vi "Take_Mass_Sequence-Sequence.vi"() -> ()   [LabVIEW 2013]
uses:
  libtiepie.dll
panel:
  in  "ConfiguredLaserCom":refnum<visa-resource-name>
  in  "Coil_angle step":dbl
  in  "Coil_radius step":dbl
  out "PlatformYCoil":dbl[](array[numeric])
  out "PlatformXCoil":dbl[](array[numeric])
  in  "AccumsPerCertify":u16=100
  out "PlatformY":dbl[](array[numeric])
  out "PlatformX":dbl[](array[numeric])
  in  "Stop":bool
  in  "ShotsPerEvalua":u16=100
  in  "Mass/Time":bool
  out "TenAccumulate":cluster{"MassX":dbl[], "TenScans":sgl[]}(graph)
  out "MassX":dbl[](array[numeric])
  out "TimeX":dbl[](array[numeric])
  out "PresentShot":i32
  out "Intensity_Total":sgl[](array[numeric])
  out "Intensity_SinglePoint":sgl[](array[numeric])
  out "InitializeCardErr":errorcluster
  in  "Record Length/Samples":u64=50000
  out "TpDeviceHandle_t":u32
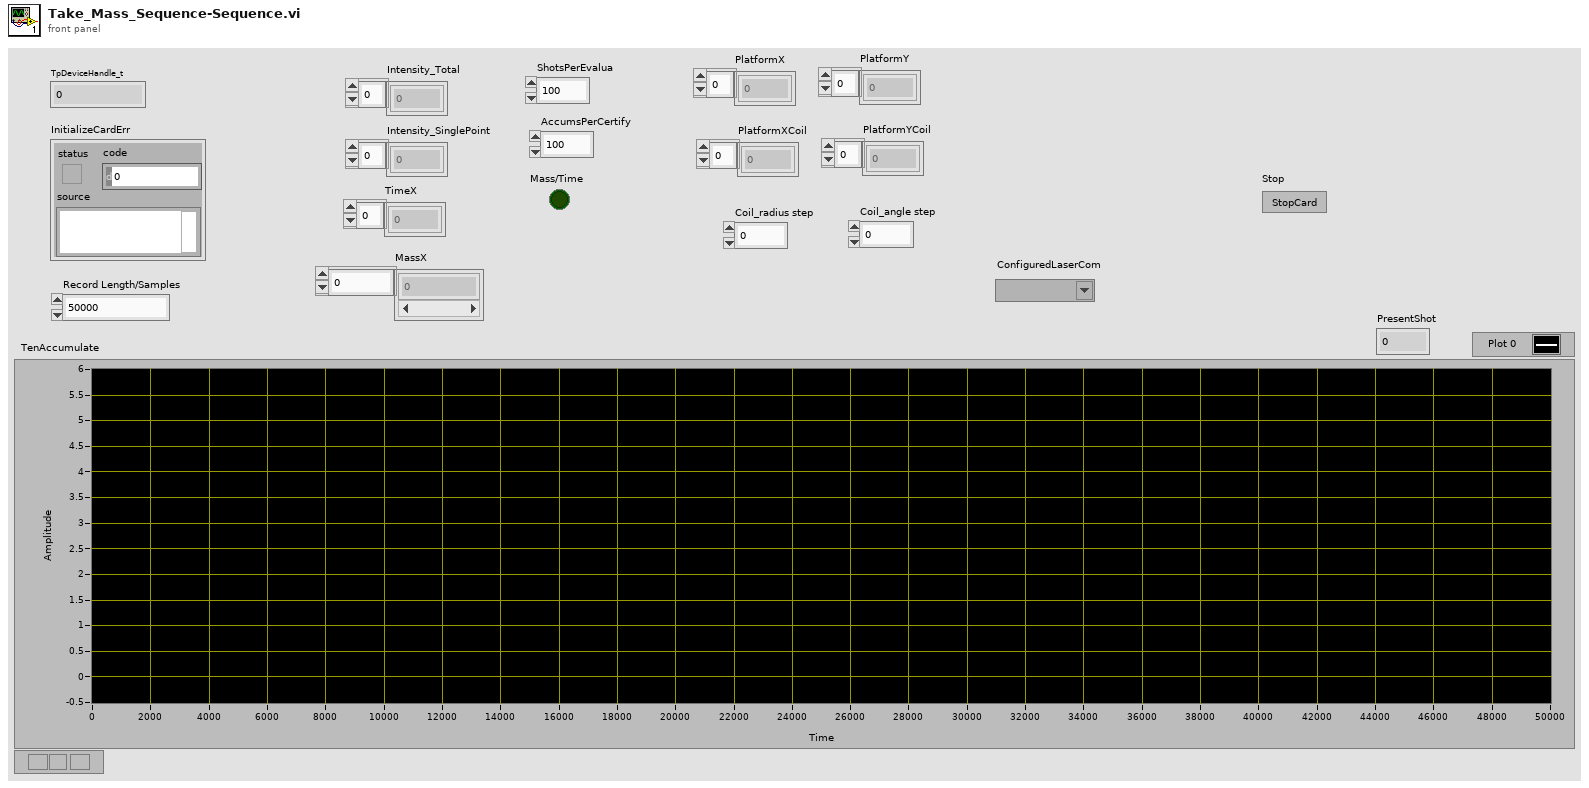
[diagram p1: front panel]
types:
  T1 = cluster{"MassX":dbl[], "Intensity_SinglePoint":sgl[]}
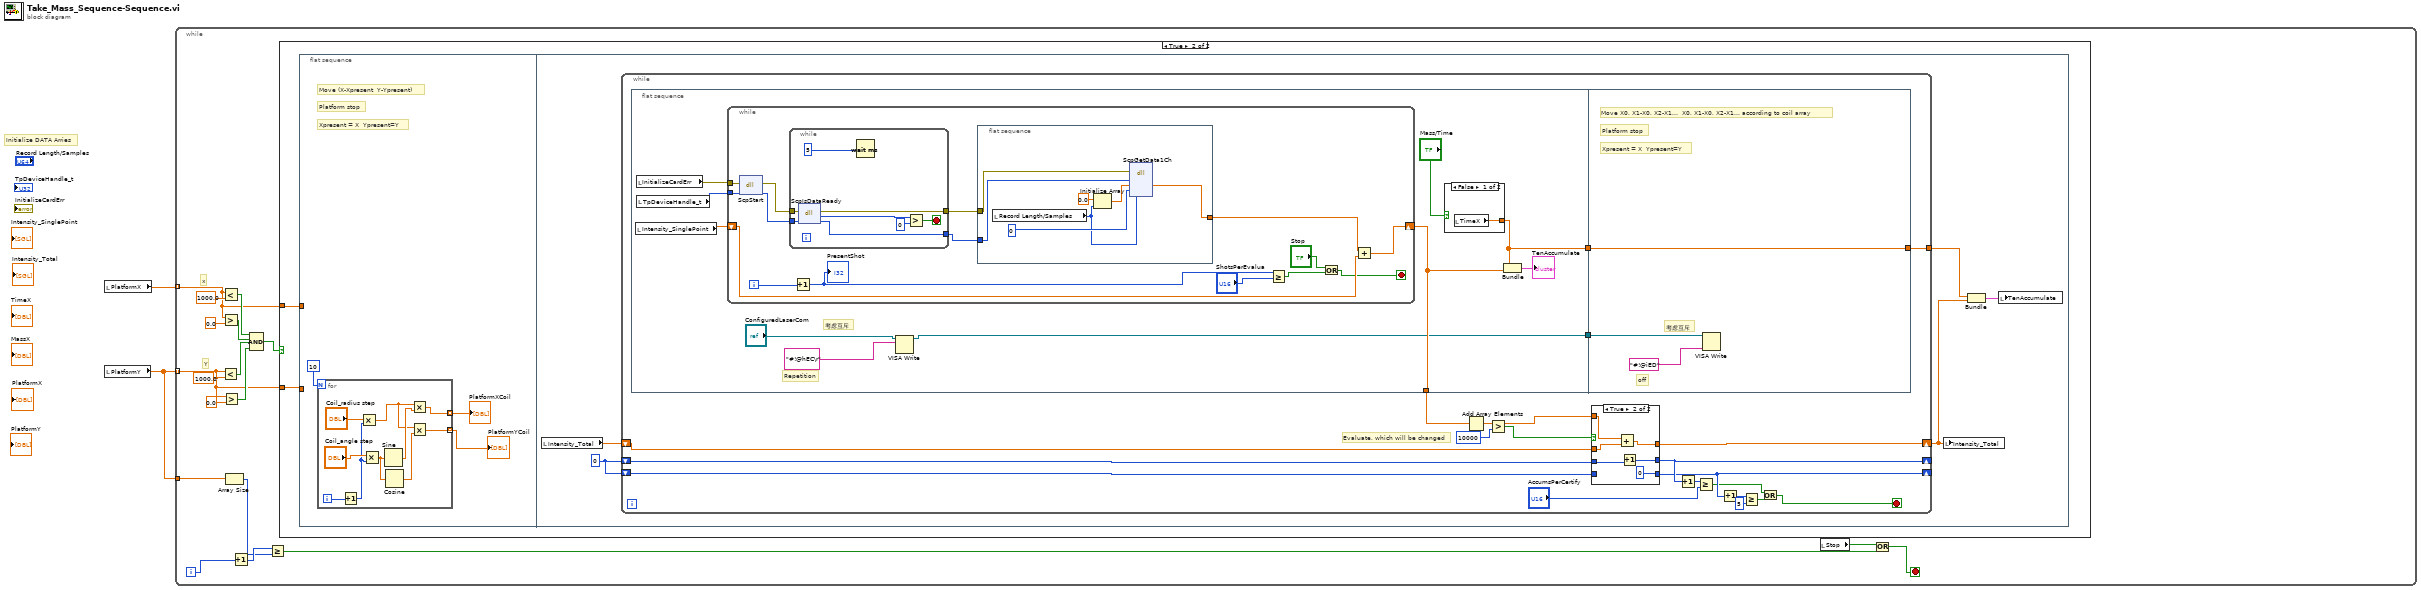
[diagram p0: block diagram]
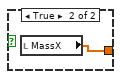
[diagram p3: hidden frame]
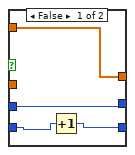
[diagram p4: hidden frame]
diagram:
  # "Initialize DATA Arries"
  n1 = local read "PlatformX"() -> (w2:dbl[])
  n2 = local read "PlatformY"() -> (w1:dbl[])
  n3 = while {
    tunnel: w2 -> [w4] mode=indexing
    tunnel: w1 -> [w3] mode=indexing
    tunnel: w1 -> [w12]
    i -> [w11]
    stop <- w6 stop-if-true
    # "Y"
    # "x"
    n4 = Less?(x=w3, y=1000.0) -> (x < y?=w14:bool)
    n5 = Less?(x=w4, y=1000.0) -> (x < y?=w16:bool)
    n6 = Greater?(x=w4, y=0.0) -> (0:w15:bool)
    n7 = Greater?(x=w3, y=0.0) -> (0:w13:bool)
    n8 = Array Size(array=w12) -> (size(s)=w9:i32)
    n9 = Increment(x=w11) -> (x+1=w10:i32)
    n10 = Compound Arithmetic op=AND(w16, w15, w14, w13) -> (w5:bool)
    n11 = Greater Or Equal?(x=w10, y=w9) -> (x >= y?=w7:bool)
    n12 = case shown="True" w5 {
      tunnel: w4 -> [_ w22]
      tunnel: w3 -> [_ w21]
      frame False {
      }
      frame True {
        n13 = flat-sequence {
          tunnel: w22 -> [_]
          tunnel: w21 -> [_]
          frame #0 {
            # "Xpresent = X  Ypresent=Y"
            # "Platform stop"
            # "Move (X-Xpresent  Y-Ypresent)"
            n14 = for {
              N: 10 -> [_]
              tunnel: [w27] -> w25 mode=indexing
              tunnel: [w26] -> w24 mode=indexing
              i -> [w35]
              n15 = Increment(x=w35) -> (x+1=w32:i32)
              n16 = Multiply(x="Coil_radius step", y=w32) -> (x*y=w28:dbl)
              n17 = Multiply(x="Coil_angle step", y=w32) -> (x*y=w31:dbl)
              n18 = Sine(x=w31) -> (sin(x)=w30:dbl)
              n19 = Cosine(x=w31) -> (cos(x)=w29:dbl)
              n20 = Multiply(x=w28, y=w30) -> (x*y=w27:dbl)
              n21 = Multiply(x=w28, y=w29) -> (x*y=w26:dbl)
            }
            "PlatformXCoil" <- w25
            "PlatformYCoil" <- w24
          }
          frame #1 {
            w39 = 0
            n22 = local read "Intensity_Total"() -> (w40:sgl[])
            n23 = while {
              shift-right: [w54] -> w37
              shift-left: w40 -> [w57]
              shift-right: [w52] -> _
              shift-left: w39 -> [w55]
              shift-right: [w49] -> _
              shift-left: w39 -> [w53]
              tunnel: [w41] -> w38
              stop <- w44 stop-if-true
              # "Evaluate, which will be changed"
              n24 = flat-sequence {
                tunnel: [w65] -> w56
                tunnel: [w62] -> w43
                tunnel: [w61] -> w42
                tunnel: w43 -> [w104]
                tunnel: [w103] -> w41
                tunnel: w42 -> [w103]
                frame #0 {
                  # "考虑互斥"
                  # "Repetition"
                  n25 = local read "Intensity_SinglePoint"() -> (w70:sgl[])
                  n26 = local read "InitializeCardErr"() -> (w67:errorcluster)
                  n27 = local read "TpDeviceHandle_t"() -> (w66:u32)
                  n28 = while {
                    tunnel: w67 -> [w87]
                    tunnel: w66 -> [w86]
                    shift-right: [w81] -> w65
                    shift-left: w70 -> [w82]
                    i -> [w80]
                    stop <- w73 stop-if-true
                    n29 = dll-call lib="PTH1Fabs CUsers82158DesktopTOF software\t数据卡\nlibtiepie.dll" fn="ScpStart"(error in=w87, "TpDeviceHandle_t"=w86) -> (error out=w85:errorcluster, "TpDeviceHandle_t"=w84:u32)  [unwired: 3 in, 1 out]
                    n30 = while {
                      tunnel: w85 -> [w95]
                      tunnel: w84 -> [w94]
                      tunnel: [w93] -> w77
                      tunnel: [w92] -> w76
                      stop <- w89 stop-if-true
                      n31 = dll-call lib="PTH1Fabs CUsers82158DesktopTOF software\t数据卡\nlibtiepie.dll" fn="ScpIsDataReady"(error in=w95, "TpDeviceHandle_t"=w94) -> (error out=w93:errorcluster, "DataReady"=w90:u8, "TpDeviceHandle_t"=w92:u32)  [unwired: 2 in, 1 out]
                      n32 = Wait (ms)(milliseconds to wait=u32 5) -> ()  [unwired: 1 out]
                      n33 = Greater?(x=w90, y=0 ("index")) -> (0:w89:bool)
                    }
                    n34 = Increment(x=w80) -> (x+1=w79:i32)
                    "PresentShot" <- w79
                    n35 = flat-sequence {
                      tunnel: [w100] -> w83
                      tunnel: w77 -> [w97]
                      tunnel: w76 -> [w96]
                      frame #0 {
                        n36 = local read "Record Length/Samples"() -> (w98:u64)
                        n37 = Initialize Array(0.0 ("element"), w98) -> (w102:dbl[])
                        n38 = dll-call lib="PTH1Fabs CUsers82158DesktopTOF software\t数据卡\nlibtiepie.dll" fn="ScpGetData1Ch"(error in=w97, "TpDeviceHandle_t"=w96, "pBufferCh1"=w102, "qwStartIndex"=u64 0, "qwSampleCount"=w98) -> ("pBufferCh1"=w100:sgl[])  [unwired: 6 in, 2 out]
                      }
                    }
                    n39 = Greater Or Equal?(x=w79, y="ShotsPerEvalua") -> (x >= y?=w74:bool)
                    n40 = Or(x="Stop", y=w74) -> (x .or. y?=w73:bool)
                    n41 = Add(x=w83, y=w82) -> (x+y=w81:sgl[])
                  }
                  n42 = VISA Write(VISA resource name="ConfiguredLaserCom", write buffer="#!@hEC\r") -> (VISA resource name out=w62:refnum<visa-resource-name>)  [unwired: 1 in, 2 out]
                  n43 = case shown="False" "Mass/Time" {
                    tunnel: [w71 w72] -> w61
                    frame False {
                      n44 = local read "TimeX"() -> (w71:dbl[])
                    }
                    frame True {
                      n45 = local read "MassX"() -> (w72:dbl[])
                    }
                  }
                  n46 = Bundle("MassX"=w61, "Intensity_SinglePoint"=w65) -> (→"TenAccumulate":T1)  [unwired: 1 in]
                }
                frame #1 {
                  # "考虑互斥"
                  # "off"
                  # "Xpresent = X  Ypresent=Y"
                  # "Platform stop"
                  # "Move X0, X1-X0, X2-X1...  X0, X1-X0, X2-X1... according to coil array"
                  n47 = VISA Write(VISA resource name=w104, write buffer="#!@iED") -> ()  [unwired: 1 in, 3 out]
                }
              }
              n48 = Add Array Elements(numeric array=w56) -> (sum=w60:sgl)
              n49 = Greater?(x=w60, y=10000) -> (0:w58:bool)
              n50 = case shown="True" w58 {
                tunnel: w57 -> [_ w115]
                tunnel: w56 -> [w108 w114]
                tunnel: w55 -> [w109 w113]
                tunnel: [w109 w112] -> w52
                tunnel: [w108 w111] -> w54
                tunnel: w53 -> [w107 _]
                tunnel: [w106 0] -> w49
                frame False {
                  n51 = Increment(x=w107) -> (x+1=w106:i32)
                }
                frame True {
                  n52 = Add(x=w114, y=w115) -> (x+y=w111:sgl[])
                  n53 = Increment(x=w113) -> (x+1=w112:i32)
                }
              }
              n54 = Increment(x=w52) -> (x+1=w51:i32)
              n55 = Greater Or Equal?(x=w51, y="AccumsPerCertify") -> (x >= y?=w45:bool)
              n56 = Increment(x=w49) -> (x+1=w48:i32)
              n57 = Greater Or Equal?(x=w48, y=5) -> (x >= y?=w46:bool)
              n58 = Or(x=w45, y=w46) -> (x .or. y?=w44:bool)
            }
            n59 = local write "Intensity_Total"(w37) -> ()
            n60 = Bundle("MassX"=w38, "Intensity_Total"=w37) -> (w36:cluster{"MassX":dbl[], "Intensity_Total":sgl[]})  [unwired: 1 in]
            n61 = local write "TenAccumulate"(w36) -> ()
          }
        }
      }
    }
    n62 = local read "Stop"() -> (w8:bool)
    n63 = Or(x=w8, y=w7) -> (x .or. y?=w6:bool)
  }
